vi "Parse Parameters Body.vi"(8 "error in (no error)":errorcluster, 11 "Body":string) -> (0 "error out":errorcluster, 3 "Body Parameters":T1[](array[typedef]))   [LabVIEW 2011, in "i3-oauth.lvlib"]
uses:
  i3-oauth.lvlib
  Controls/key-value-pairs.ctl
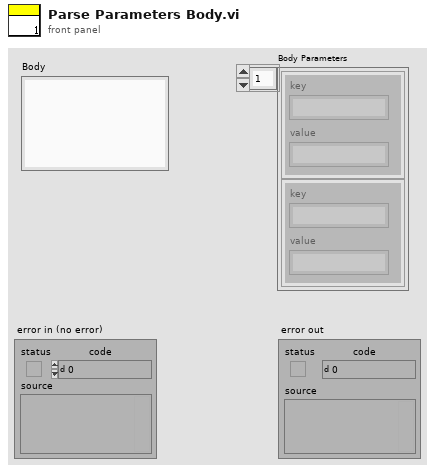
[diagram p1: front panel]
types:
  T1 = typedef "i3-oauth.lvlib/key-value-pairs.ctl" = cluster{"key":string, "value":string}
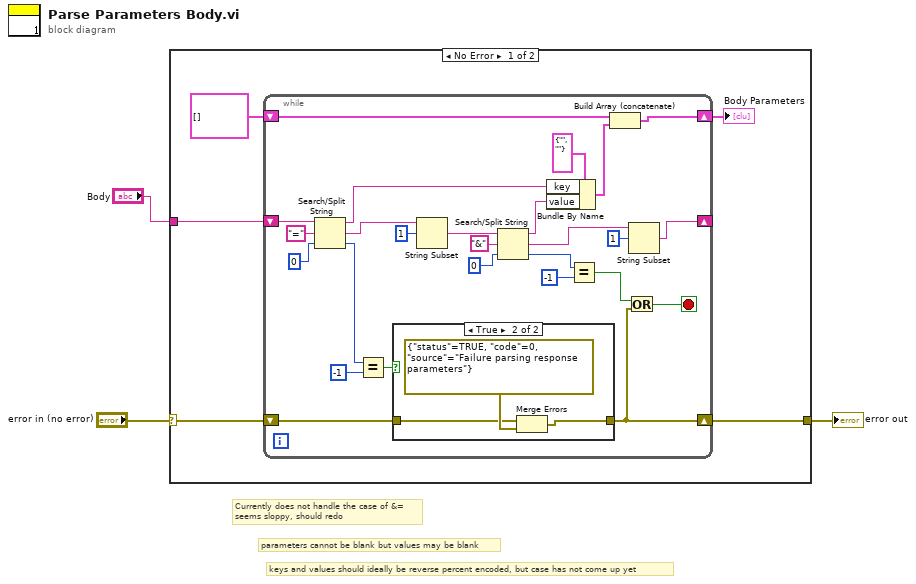
[diagram p0: block diagram]
diagram:
  # "keys and values should ideally be reverse percent encoded, but case has not come up yet"
  # "parameters cannot be blank but values may be blank"
  # "Currently does not handle the case of &=\nseems sloppy, should redo"
  n1 = case shown="No Error" "error in (no error)" {
    selector: "error in (no error)" -> [w5 w39]
    tunnel: "Body" -> [w8 _]
    tunnel: [w4 w39] -> w1
    frame No Error {
      n2 = while {
        shift-right: [w26] -> w6
        shift-left: T1[] [] ("Body Parameters") -> [w28]
        shift-right: [w9] -> w4
        shift-left: w5 -> [w10]
        shift-right: [w13] -> _
        shift-left: w8 -> [w33]
        stop <- w21 stop-if-true
        n3 = Search/Split String(string=w33, search string/char (-)="=", offset (0)=0) -> (substring before match=w31:string, match + rest of string=w20:string, offset of match=w23:i32)
        n4 = Equal?(x=w23, y=-1) -> (x = y?=w11:bool)
        n5 = case shown="True" w11 {
          tunnel: w10 -> [w35 w37]
          tunnel: [w35 w36] -> w9
          frame False {
          }
          frame True {
            n6 = Merge Errors(w37, errorcluster {"status"=TRUE, "code"=0, "source"="Failure parsing response parameters"} ("error in (no error)")) -> (w36:errorcluster)
          }
        }
        n7 = String Subset(string=w20, offset (0)=1) -> (substring=w19:string)  [unwired: 1 in]
        n8 = Search/Split String(string=w19, search string/char (-)="&", offset (0)=0) -> (substring before match=w15:string, match + rest of string=w12:string, offset of match=w25:i32)
        n9 = Bundle By Name(cluster=T1 {"key"="", "value"=""} ("Key Value Pair"), "key"=w31, "value"=w15) -> (w27:T1)
        n10 = Equal?(x=w25, y=-1) -> (x = y?=w22:bool)
        n11 = Build Array (concatenate)(w28, w27) -> (w26:T1[])
        n12 = Or(x=w22, y=w9) -> (x .or. y?=w21:bool)
        n13 = String Subset(string=w12, offset (0)=1) -> (substring=w13:string)  [unwired: 1 in]
      }
      "Body Parameters" <- w6
    }
    frame Error {
    }
  }
  "error out" <- w1
